vi "Close.vi"(8 "error in (no error)":errorcluster, 11 "CCD in":refnum<class "Motor.lvclass">) -> (0 "error out":errorcluster, 3 "CCD out":refnum<class "Motor.lvclass">)   [LabVIEW 2016, in "Hardware.lvlib" / "Motor.lvlib" / "Motor.lvclass"]
uses:
  <userlib>/Common Components/Hardware/Motor/Motor/Motor.lvclass
  <userlib>/Common Components/Hardware/Motor/Motor/Motor.lvclass/Motor.ctl
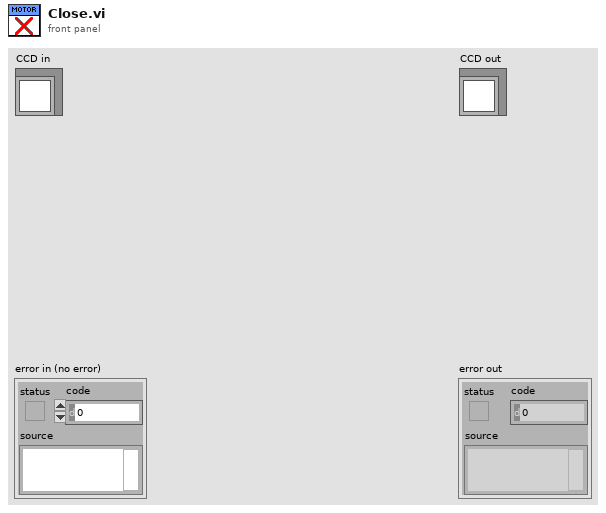
[diagram p1: front panel]
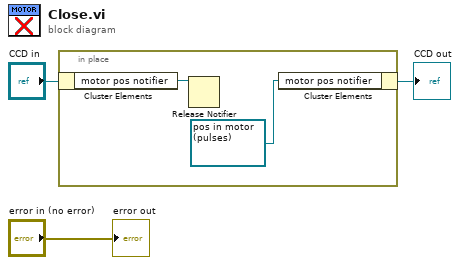
[diagram p0: block diagram]
diagram:
  n1 = in-place {
    n2 = in-place-cluster #1("CCD in") -> ("motor pos notifier"=w5:refnum<notifier>)
    n3 = Release Notifier(notifier=w5) -> ()  [unwired: 2 in, 3 out]
    n4 = in-place-cluster #1("motor pos notifier"=refnum<notifier> refnum) -> (→"CCD out":refnum<class "Motor.lvclass">)
  }
  "error out" <- "error in (no error)"
